vi "Get Column Config.vi"(8 "error in (no error)":errorcluster, 11 "Ctrl Refnum Column in":refnum<class "Ctrl Refnum Column.lvclass">) -> (0 "error out":errorcluster, 2 "Column Configuration":refnum<class "Column Configuration.lvclass">, 3 "Ctrl Refnum Column out":refnum<class "Ctrl Refnum Column.lvclass">)   [LabVIEW 2020, in "Basic Fields.lvlib" / "Ctrl Refnum Column.lvclass"]
uses:
  Ctrl Refnum Column.lvclass
  Column Interface/Column Configuration Interface Class/Column Configuration.lvclass
  Ctrl Refnum Column.lvclass/Ctrl Refnum Column.ctl
  Basic Columns/Basic Columns/Column Class/Column Parent.lvclass
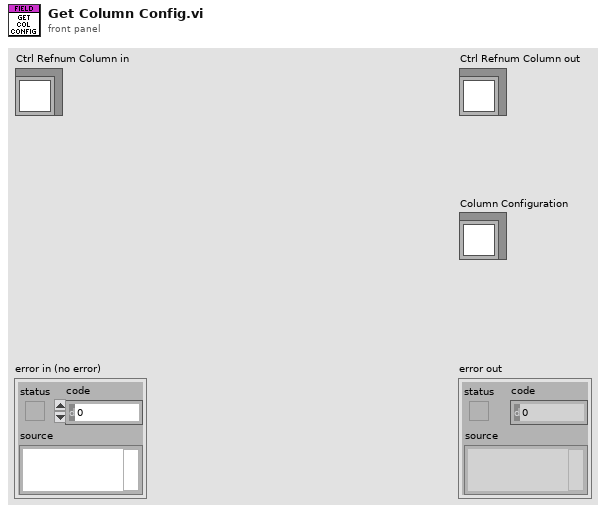
[diagram p1: front panel]
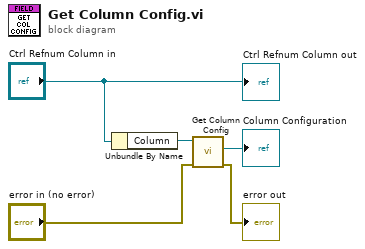
[diagram p0: block diagram]
diagram:
  n1 = Unbundle By Name("Ctrl Refnum Column in") -> ("Column"=w4:refnum<class "Column Parent.lvclass">)
  n2 = call-dynamic "Get Column Config.vi"("error in (no error)"="error in (no error)", "Column Parent in"=w4) -> ("error out"=→"error out":errorcluster, "Column Configuration"=→"Column Configuration":refnum<class "Column Configuration.lvclass">)  [unwired: 7 in, 1 out]
  "Ctrl Refnum Column out" <- "Ctrl Refnum Column in"
